vi "Set EL Mode.vi"(7 "el_logicEL":T2(ring), 8 "error in (no error)":errorcluster, 9 "el_modeEL":T1(ring), 10 "el_enableEL":T3(ring), 11 "Motor in":refnum<class "Motor.lvclass">) -> (0 "error out":errorcluster, 3 "Motor out":refnum<class "Motor.lvclass">)   [LabVIEW 2016, in "Hardware.lvlib" / "Motor.lvlib" / "Motor.lvclass"]
uses:
  <userlib>/Common Components/Hardware/Motor/Motor/Motor.lvclass
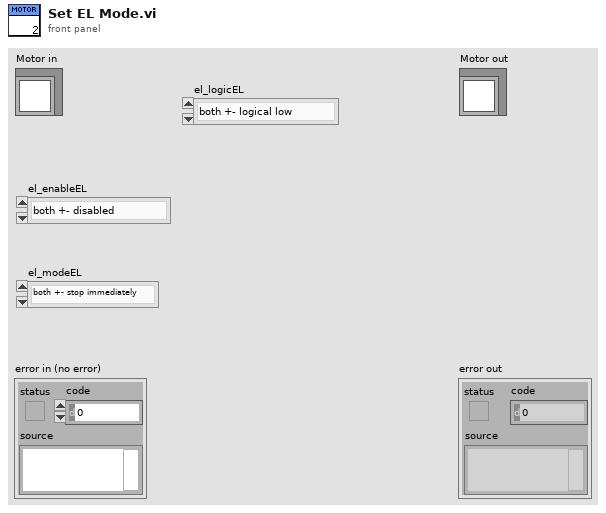
[diagram p1: front panel]
types:
  T1 = enum16{"both +- stop immediately", "both +- decelerate to stop", "+ stop immediately, - decelerate to stop", "+ decelerate to stop, - stop immediately"}
  T2 = enum16{"both +- logical low", "both +- logical high", "+ logical low, - logical high", "+ logical high, - logical low"}
  T3 = enum16{"both +- disabled", "both +- enabled", "+ disabled, - enabled", "+ enabled, - disabled"}
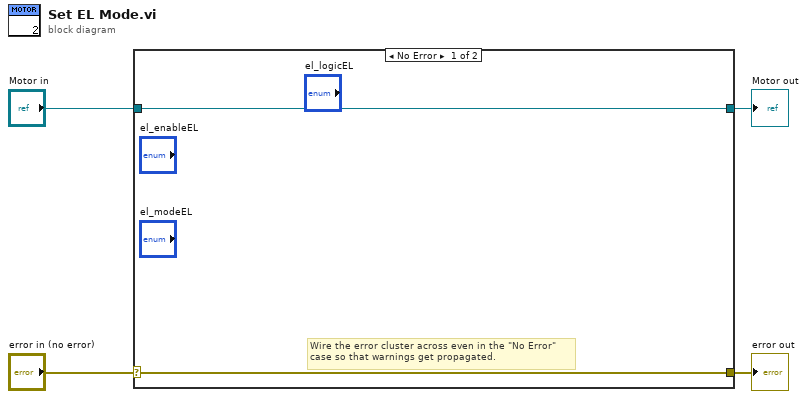
[diagram p0: block diagram]
diagram:
  n1 = case shown="No Error" "error in (no error)" {
    selector: "error in (no error)" -> [w5 w8]
    tunnel: [w5 w8] -> w3
    tunnel: [w6 w7] -> w1
    tunnel: "Motor in" -> [w6 w7]
    frame No Error {
      # "Wire the error cluster across even in the \"No Error\"\ncase so that warnings get propagated."
    }
    frame Error {
    }
  }
  "error out" <- w3
  "Motor out" <- w1
